vi "Main.vi"   [LabVIEW 2024]
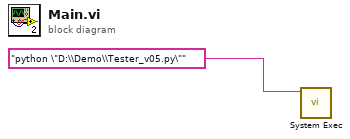
[diagram p0: block diagram]
diagram:
  n1 = call <vilib>:"System Exec.vi"("command line"="python \"D:\\Demo\\Tester_v05.py\"") -> ()  [unwired: 7 in, 4 out]
